vi "Polynomial_convert.vi"(3 "Calib constants":dbl[](array[numeric])=[0.2727, 22.328, 22.281, -22.056, 13.889] format="%.3e", 6 "Voltage":dbl format="%.3f") -> (1 "Eng Values":dbl format="%.2f")   [LabVIEW 2011]
panel:
  # "x^0\nx^1\nx^2\nx^3\nx^4"
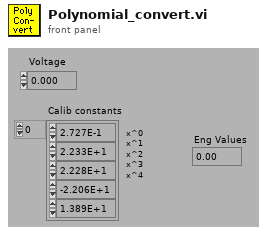
[diagram p1: front panel]
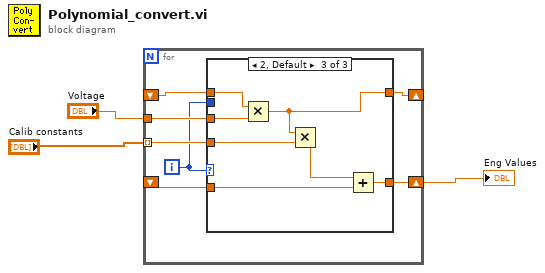
[diagram p0: block diagram]
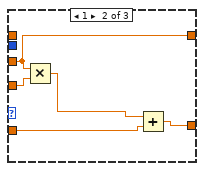
[diagram p3: hidden frame]
diagram:
  n1 = for {
    shift-right: [w7] -> w2
    shift-left: _ -> [w8]
    tunnel: "Voltage" -> [w10]
    tunnel: "Calib constants" -> [w9] mode=indexing
    shift-right: [w5] -> _
    shift-left: _ -> [w4]
    i -> [w6]
    n2 = case shown="2, Default" w6 {
      tunnel: w6 -> [_ _ _]
      tunnel: w10 -> [_ w13 w20]
      tunnel: w9 -> [w12 w17 w24]
      tunnel: w8 -> [_ w15 w22]
      tunnel: [w12 w16 w21] -> w7
      tunnel: [w11 w13 w18] -> w5
      tunnel: w4 -> [w11 _ w19]
      frame 0 {
      }
      frame 1 {
        n3 = Multiply(x=w13, y=w17) -> (x*y=w14:dbl)
        n4 = Add(x=w14, y=w15) -> (x+y=w16:dbl)
      }
      frame 2, Default {
        n5 = Multiply(x=w19, y=w20) -> (x*y=w18:dbl)
        n6 = Multiply(x=w18, y=w24) -> (x*y=w23:dbl)
        n7 = Add(x=w23, y=w22) -> (x+y=w21:dbl)
      }
    }
  }
  "Eng Values" <- w2
